vi "Evaluate.vi"(8 "error in (no error)":errorcluster, 10 "Point":dbl[](array[numeric]), 11 "PassObjective in":refnum<class "PassObjective.lvclass">) -> (0 "error out":errorcluster, 2 "Evaluation":dbl, 3 "PassObjective out":refnum<class "PassObjective.lvclass">)   [LabVIEW 2023, in "PassObjective.lvclass"]
uses:
  PassObjective.lvclass
  Utilities_class/Utilities.lvclass
  Team_class/OffensivePlay.ctl
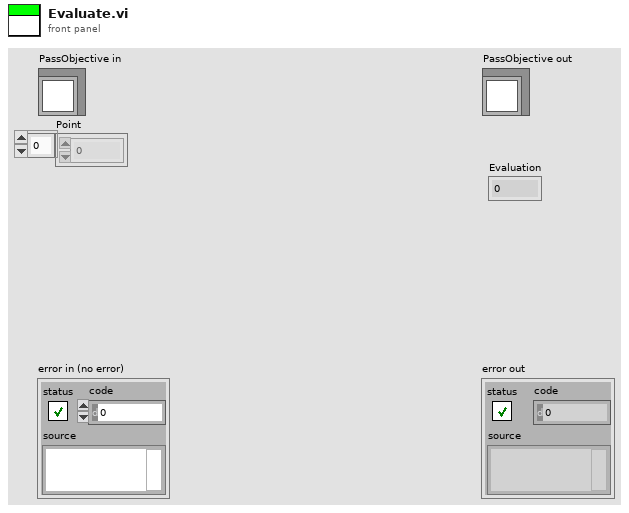
[diagram p1: front panel]
types:
  T1 = typedef "OffensivePlay.ctl" = enum16{"5RobotsPassGamePlay", "5PreparePassGame", "5RobotsKeeperGame", "KeeperPassToStriker", "5RobotsNormalGamePlay", "PrepareKeeperPass", "ACBPass", "ABCPass", "PrepareTriplePass", "TableWithStriker", "TableWith2ndStrikerPlay", "PrepareDoublePass", "PrepareRollToPass", "SimplePass", "PreparePass", "PassToStriker", "BallOutOfField", "PassTo2ndStriker", "StopOffensive", "Prepare Penalty Enemy", "EnemyPossessionAtEnemyField", "EnemyPossesionAtOurField", "TestPlay", "PreparePenaltyAlly", "KickPenaltyAlly", "PrepareKickoffAlly", "PrepareKickoffEnemy", "IndirectEnemy", "DirectEnemy", "PreparePassInGame1", "NormalGame", "DirectKick", "Pass", "Halt", "Timeout", "PassPlay", "PenaltyEnemy"}
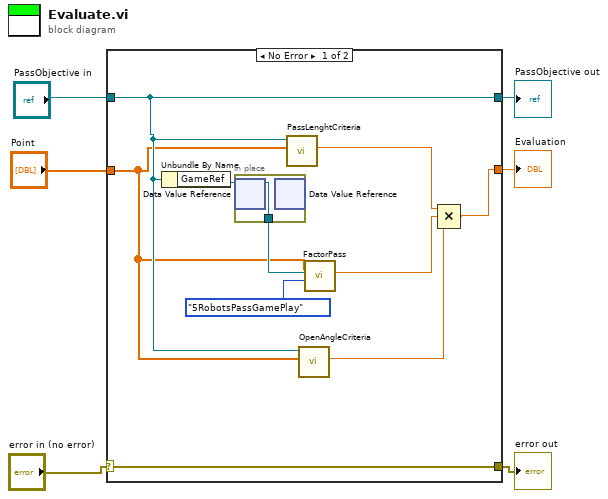
[diagram p0: block diagram]
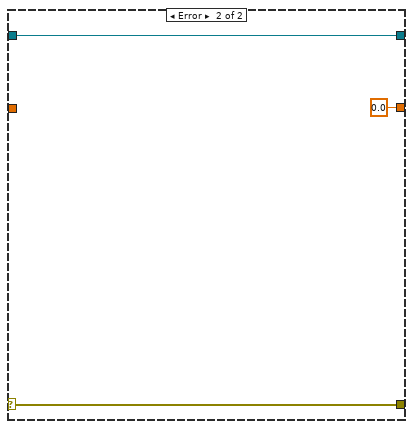
[diagram p2: hidden frame]
diagram:
  n1 = case shown="No Error" "error in (no error)" {
    selector: "error in (no error)" -> [w16 w20]
    tunnel: [w16 w20] -> w5
    tunnel: "PassObjective in" -> [w10 w19]
    tunnel: [w10 w19] -> w3
    tunnel: "Point" -> [w9 _]
    tunnel: [w7 0.0 ("evaluation")] -> w1
    frame No Error {
      n2 = Unbundle By Name(w10) -> ("GameRef"=w15:refnum<data-value>)
      n3 = in-place {
        in-place-border: [w17] -> w11
        n4 = in-place-dvr #1(w15) -> (w17:refnum<class "Game.lvclass">)  [unwired: 1 out]
        n5 = in-place-dvr #1() -> ()  [unwired: 1 in, 2 out]
      }
      n6 = call-dynamic "PassLenghtCriteria.vi"("Point"=w9, "PassObjective in"=w10) -> ("Evaluation"=w13:dbl)  [unwired: 7 in, 2 out]
      n7 = call-dynamic "OpenAngleCriteria.vi"("point"=w9, "PassObjective in"=w10) -> ("evaluation"=w8:dbl)  [unwired: 7 in, 2 out]
      n8 = call "FactorPass.vi"("Robot"=w9, "OffensivePlay"=OffensivePlay."5RobotsPassGamePlay", "Game"=w11) -> ("Critério de marcação Normalizado"=w12:dbl)  [unwired: 6 in, 2 out]
      n9 = Compound Arithmetic op=MULTIPLY(w13, w12, w8) -> (w7:dbl)
    }
    frame Error {
    }
  }
  "error out" <- w5
  "PassObjective out" <- w3
  "Evaluation" <- w1
